vi "Append VI Hierarchy to Report.vi"   [LabVIEW 2017, in "NI_ReportGenerationCore.lvlib"]
doc: "Appends the hierarchy of the VI you specify in <B>VI</B> to a report. Wire data to the <B>VI</B> input to determine the polymorphic instance to use or manually select the instance."
uses:
  <vilib>/Utility/NIReport.llb/NI_ReportGenerationCore.lvlib
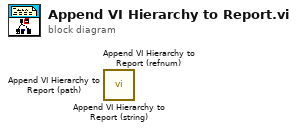
[diagram p0: block diagram]
diagram:
  n1 = call <vilib>:"Append VI Hierarchy to Report (string).vi"() -> ()  [unwired: 11 in, 5 out]
  n2 = call <vilib>:"Append VI Hierarchy to Report (refnum).vi"() -> ()  [unwired: 11 in, 5 out]
  n3 = call <vilib>:"Append VI Hierarchy to Report (path).vi"() -> ()  [unwired: 11 in, 5 out]
